vi "Partir_archivos.vi"() -> ()   [LabVIEW 2015]
panel:
  out "Array":errorcluster[](array[cluster])
  in  "Nº inductivos":i32
  in  "Nº acel":i32
  out "T, v, UT":sgl[](array[numeric])
  out "Waveform Graph":waveform(sgl)[](graph)
  in  "Folder Path":path
  out "error out":errorcluster
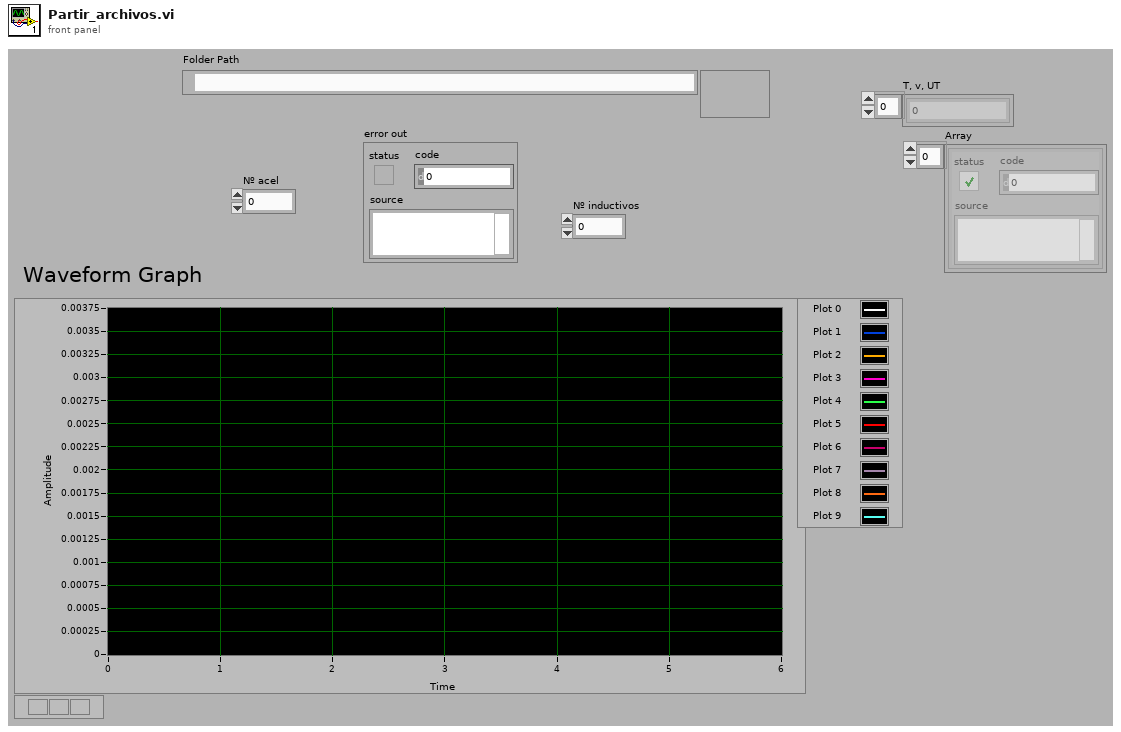
[diagram p1: front panel]
types:
  T1 = enum16{"big-endian, network order", "native, host order", "little-endian"}
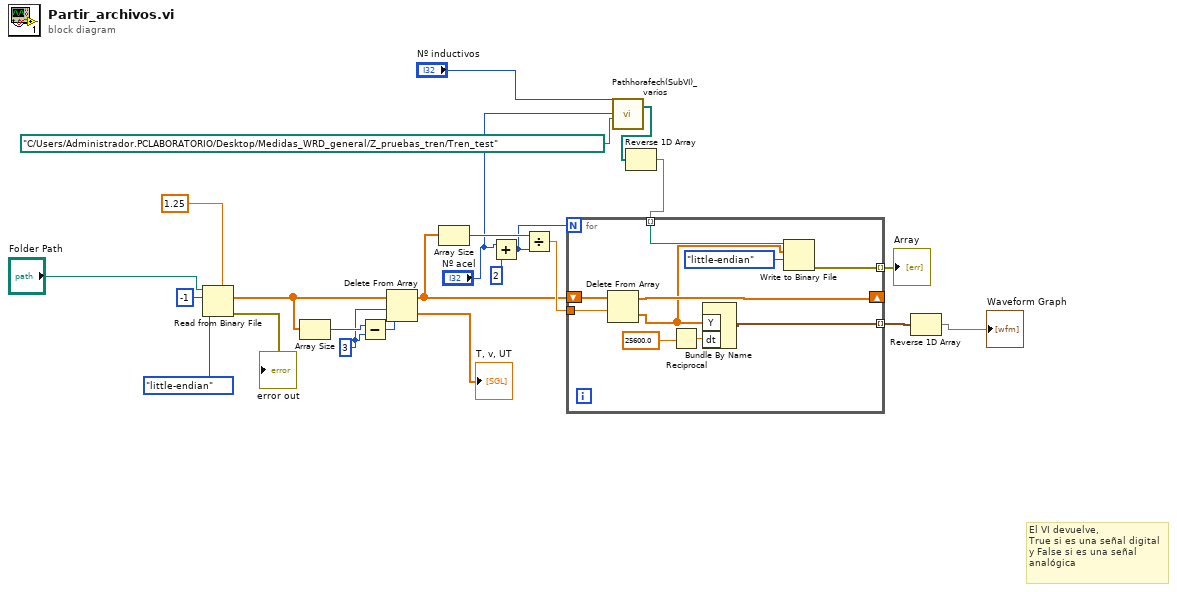
[diagram p0: block diagram]
diagram:
  w17 = 3 ("length")
  # "El VI devuelve,\nTrue si es una señal digital\ny False si es una señal\nanalógica"
  n1 = Read from Binary File(5:sgl 1.25, 9:T1."little-endian" ("byte order (0:big-endian, network order)"), 10:-1 ("count (1)"), 11:"Folder Path") -> (0:→"error out":errorcluster, 2:w16:sgl[])  [unwired: 1 in, 3 out]
  n2 = Array Size(array=w16) -> (size(s)=w19:i32)
  n3 = Subtract(x=w19, y=w17) -> (x-y=w18:i32)
  n4 = Delete From Array(array=w16, length=w17, index=w18) -> (deleted portion=→"T, v, UT":sgl[], array with subset deleted=w13:sgl[])
  n5 = Array Size(array=w13) -> (size(s)=w15:i32)
  n6 = Add(x="Nº acel", y=2) -> (x+y=w9:i32)
  n7 = Divide(x=w15, y=w9) -> (x/y=w14:dbl)
  n8 = call "Pathhorafech(SubVI)_varios.vi"("Folder path"=path "C:/Users/Administrador.PCLABORATORIO/Desktop/Medidas_WRD_general/Z_pruebas_tren/Tren_test", "Nº de acelerómetros"="Nº acel", "Nº inductivos"="Nº inductivos") -> ("Acel_Paths"=w2:path[])  [unwired: 1 in, 1 out]
  n9 = Reverse 1D Array(array=w2) -> (reversed array=w1:path[])
  n10 = for {
    N: w9 -> [_]
    tunnel: [w33] -> w8 mode=indexing
    shift-right: [w27] -> _
    shift-left: w13 -> [w30]
    tunnel: w14 -> [w29]
    tunnel: w1 -> [w28] mode=indexing
    tunnel: [w25] -> w3 mode=indexing
    n11 = Delete From Array(array=w30, length=w29) -> (deleted portion=w24:sgl[], array with subset deleted=w27:sgl[])  [unwired: 1 in]
    n12 = Reciprocal(x=25600.0 ("dt")) -> (1/x=w31:dbl)
    n13 = Bundle By Name("Y"=w24, "dt"=w31) -> (w33:waveform(sgl))  [unwired: 1 in]
    n14 = Write to Binary File(file (use dialog)=w28, data=w24, 9:T1."little-endian" ("byte order (0:big-endian, network order)")) -> (error out=w25:errorcluster)  [unwired: 3 in, 2 out]
  }
  "Array" <- w3
  n15 = Reverse 1D Array(array=w8) -> (reversed array=→"Waveform Graph":waveform(sgl)[])
